vi "CRYSet RTA Front Panel.vi"(11 "Vi Ref in":refnum<vi> caption="Vi Ref") -> (3 "Vi Ref out":refnum<vi> caption="Vi Ref")   [LabVIEW 2013]
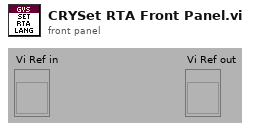
[diagram p1: front panel]
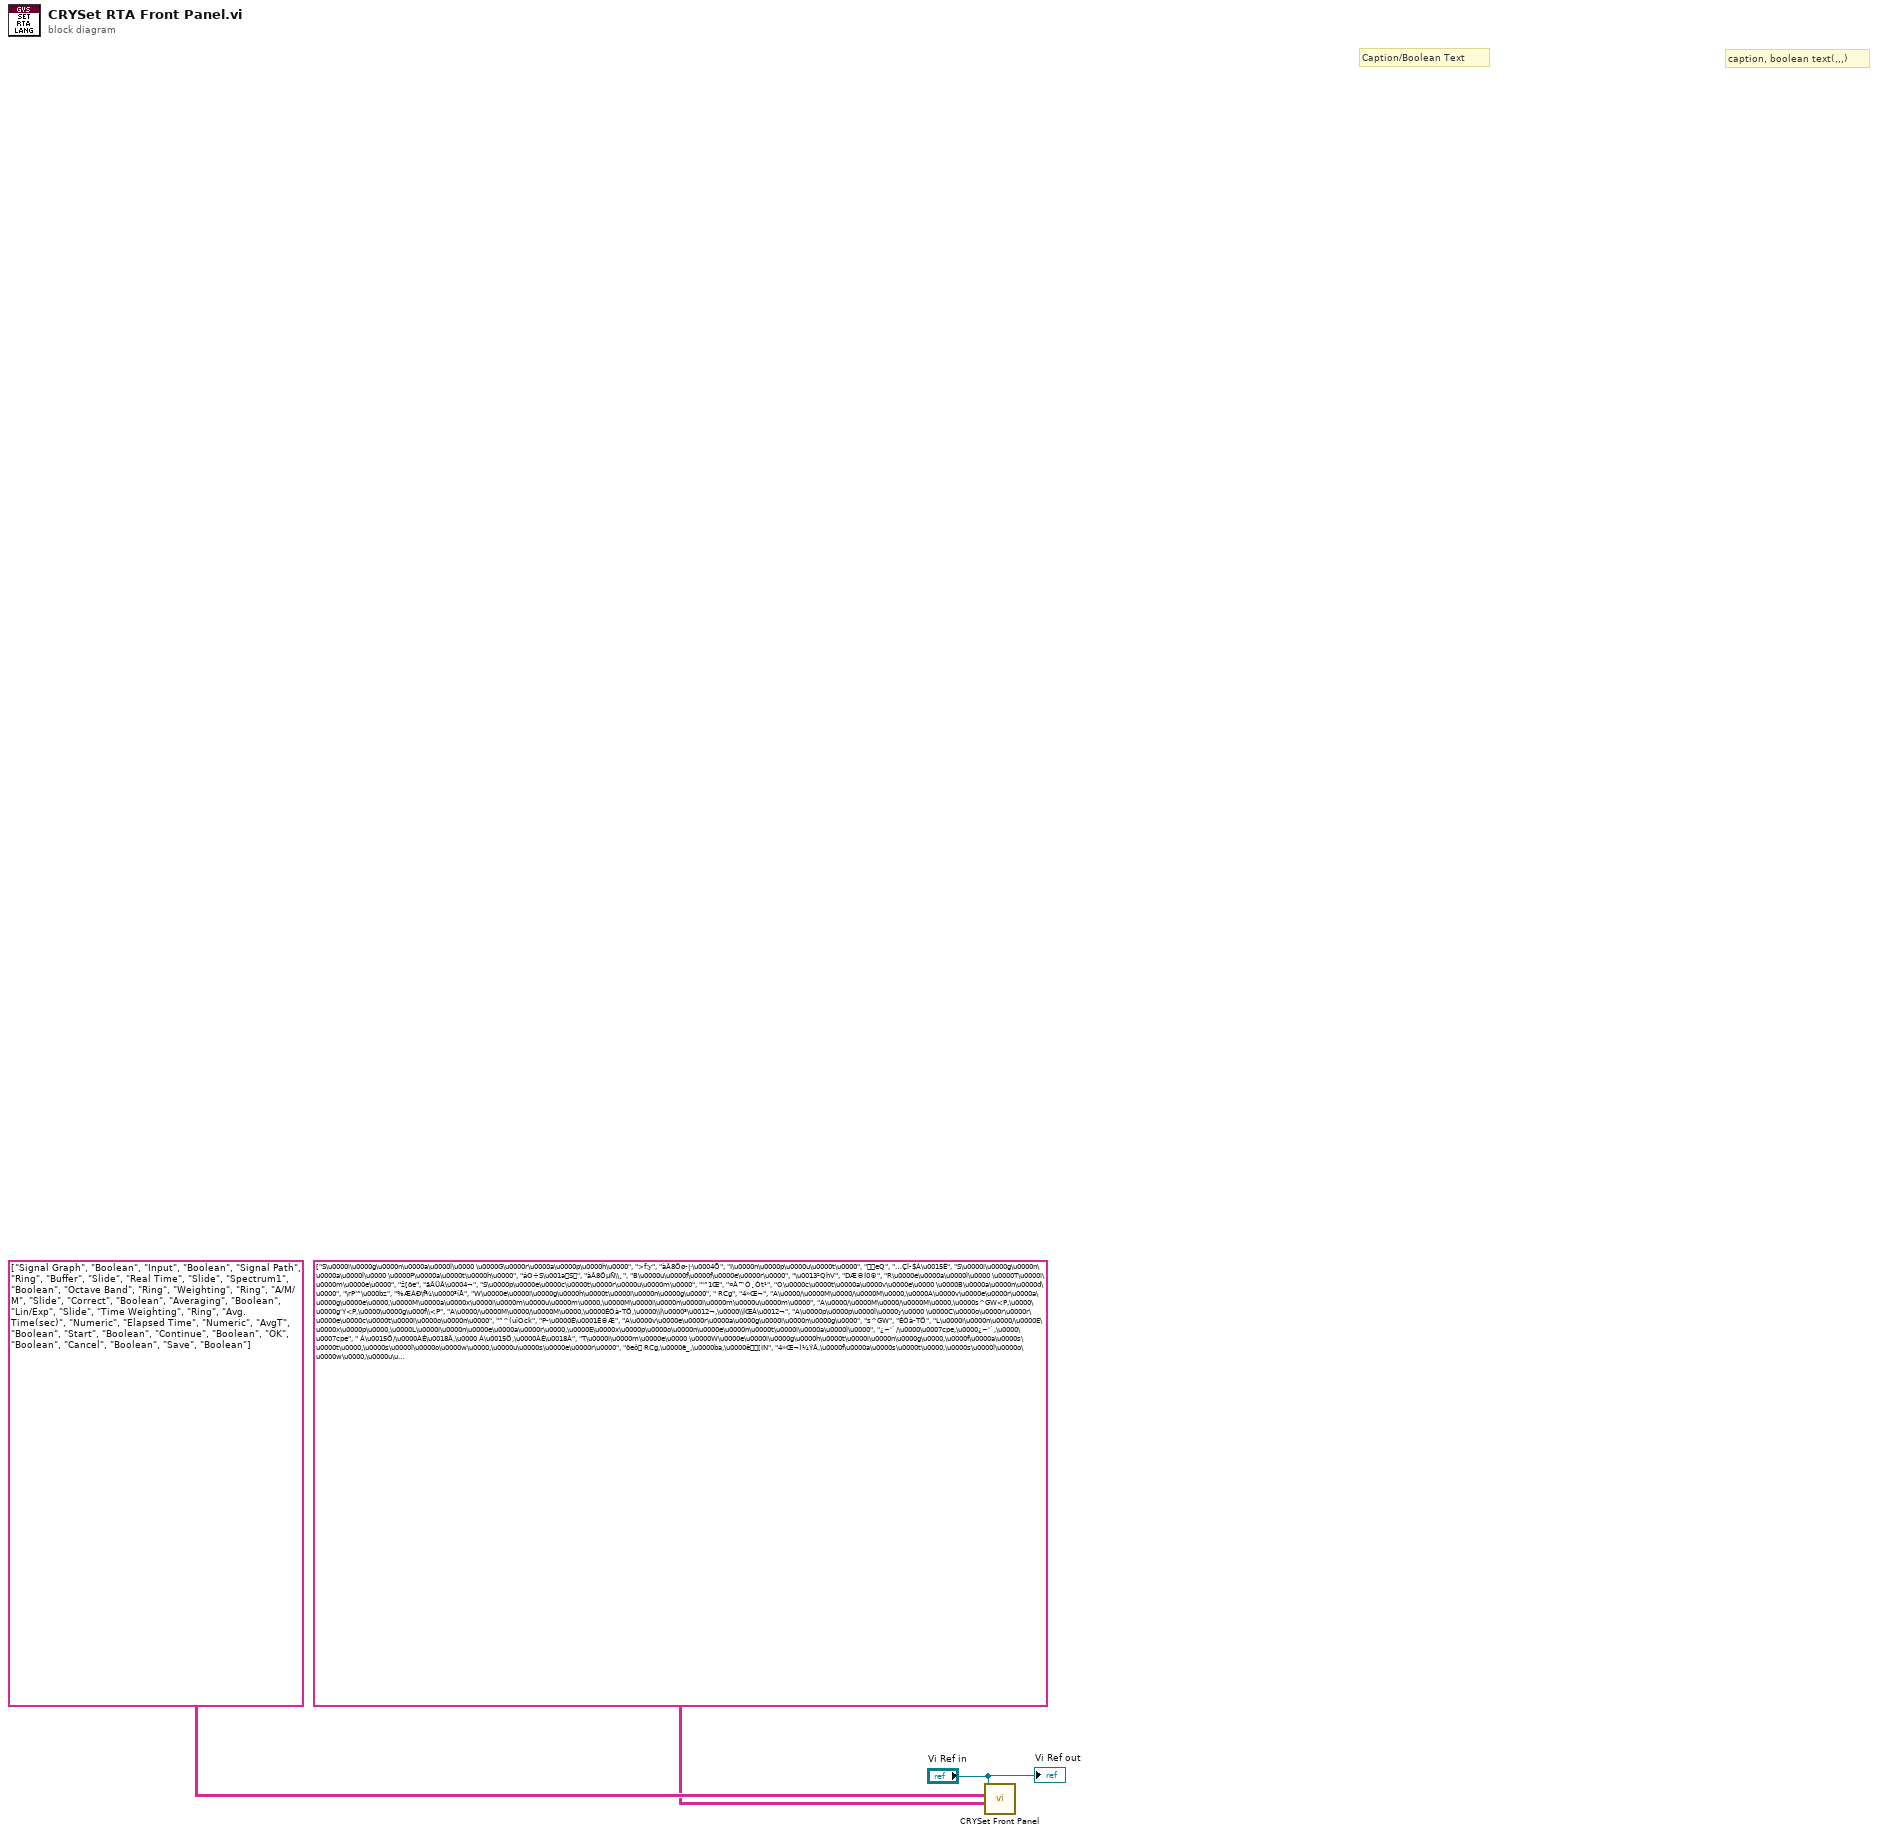
[diagram p0: block diagram]
diagram:
  # "caption, boolean text(,,,)"
  # "Caption/Boolean Text"
  n1 = call "CRYSet Front Panel.vi"("Caption(Boolean Text)"=string[][] [["S\u0000i\u0000g\u0000n\u0000a\u0000l\u0000 \u0000G\u0000r\u0000a\u0000p\u0000h\u0000", ">f:y", "àÂ8Öø­|·\u0004Õ"], ["I\u0000n\u0000p\u0000u\u0000t\u0000", "eQ", "…Çl­$Á\u0015È"], ["S\u0000i\u0000g\u0000n\u0000a\u0000l\u0000 \u0000P\u0000a\u0000t\u0000h\u0000", "áO÷S\u001aS", "àÂ8ÖµÑ\\¸"], ["B\u0000u\u0000f\u0000f\u0000e\u0000r\u0000", "\u0013²QhV", "DÆ©Í0®"], ["R\u0000e\u0000a\u0000l\u0000 \u0000T\u0000i\u0000m\u0000e\u0000", "ž[öe", "äÂÜÂ\u0004¬"], ["S\u0000p\u0000e\u0000c\u0000t\u0000r\u0000u\u0000m\u0000", "‘˜1Œ", "¤Â™Ó¸Òt¹"], ["O\u0000c\u0000t\u0000a\u0000v\u0000e\u0000 \u0000B\u0000a\u0000n\u0000d\u0000", "\rP‘˜\u000bz", "%ÆÀÐ\f¾\u0000³íÅ"], ["W\u0000e\u0000i\u0000g\u0000h\u0000t\u0000i\u0000n\u0000g\u0000", " RCg", "4»Œ¬"], ["A\u0000/\u0000M\u0000/\u0000M\u0000,\u0000A\u0000v\u0000e\u0000r\u0000a\u0000g\u0000e\u0000,\u0000M\u0000a\u0000x\u0000i\u0000m\u0000u\u0000m\u0000,\u0000M\u0000i\u0000n\u0000i\u0000m\u0000u\u0000m\u0000", "A\u0000/\u0000M\u0000/\u0000M\u0000,\u0000s^GW<P,\u0000\u0000g'Y<P,\u0000\u0000g\u000f\\<P", "A\u0000/\u0000M\u0000/\u0000M\u0000,\u0000ÉÓà­TÖ,\u0000\\Í\u0000³\u0012¬,\u0000\\ÍŒÁ\u0012¬"], ["A\u0000p\u0000p\u0000l\u0000y\u0000 \u0000C\u0000o\u0000r\u0000r\u0000e\u0000c\u0000t\u0000i\u0000o\u0000n\u0000", "”^(uîOck", "P­\u0000É\u0001È©Æ"], ["A\u0000v\u0000e\u0000r\u0000a\u0000g\u0000i\u0000n\u0000g\u0000", "s^GW", "ÉÓà­TÖ"], ["L\u0000i\u0000n\u0000/\u0000E\u0000x\u0000p\u0000,\u0000L\u0000i\u0000n\u0000e\u0000a\u0000r\u0000,\u0000E\u0000x\u0000p\u0000o\u0000n\u0000e\u0000n\u0000t\u0000i\u0000a\u0000l\u0000", "¿~'`/\u0000\u0007cpe,\u0000¿~'`,\u0000\u0007cpe", " Á\u0015Ö/\u0000ÀÉ\u0018Â,\u0000 Á\u0015Ö,\u0000ÀÉ\u0018Â"], ["T\u0000i\u0000m\u0000e\u0000 \u0000W\u0000e\u0000i\u0000g\u0000h\u0000t\u0000i\u0000n\u0000g\u0000,\u0000f\u0000a\u0000s\u0000t\u0000,\u0000s\u0000l\u0000o\u0000w\u0000,\u0000u\u0000s\u0000e\u0000r\u0000", "öeô RCg,\u0000ë_,\u0000ba,\u0000ê[IN", "4»Œ¬)¼ÝÂ,\u0000f\u0000a\u0000s\u0000t\u0000,\u0000s\u0000l\u0000o\u0000w\u0000,\u0000u\u0000s\u0000e\u0000r\u0000"], ["A\u0000v\u0000g\u0000.\u0000 \u0000T\u0000i\u0000m\u0000e\u0000(\u0000s\u0000e\u0000c\u0000)\u0000", "s^GWöeô•(\u0000Òy)\u0000", "ÉÓà­ÜÂ\u0004¬(\u0000\bÍ)\u0000"], ["E\u0000l\u0000a\u0000p\u0000s\u0000e\u0000d\u0000 \u0000T\u0000i\u0000m\u0000e\u0000", "ˆm\u0017€öeô•", "½¬ü¬ÜÂ\u0004¬"], ["A\u0000v\u0000e\u0000r\u0000a\u0000g\u0000i\u0000n\u0000g\u0000", "s^GW.\u0000.\u0000.\u0000", "ÉÓà­.\u0000.\u0000.\u0000"], ["S\u0000t\u0000a\u0000r\u0000t\u0000", "\u0000_ \u0000ËY", "ÜÂ \u0000‘Ç"], ["C\u0000o\u0000n\u0000t\u0000i\u0000n\u0000u\u0000e\u0000", "ç~ \u0000í~", "Ä¬ \u0000Á"], ["O\u0000K\u0000", "nx¤‹", "UÖxÇ"], ["C\u0000a\u0000n\u0000c\u0000e\u0000l\u0000", "ÖSˆm", "èÍŒÁ"], ["S\u0000a\u0000v\u0000e\u0000 \u0000t\u0000o\u0000 \u0000 \u0000C\u0000u\u0000r\u0000v\u0000e\u0000L\u0000i\u0000b\u0000", "ÝOX[0Ròf¿~“^", "á¬ Á\u001cÁà¬ÐÅ \u0000ô¼\u0000­"]], "Control ID and Type(Label Name, Type)"=string[][] [["Signal Graph", "Boolean"], ["Input", "Boolean"], ["Signal Path", "Ring"], ["Buffer", "Slide"], ["Real Time", "Slide"], ["Spectrum1", "Boolean"], ["Octave Band", "Ring"], ["Weighting", "Ring"], ["A/M/M", "Slide"], ["Correct", "Boolean"], ["Averaging", "Boolean"], ["Lin/Exp", "Slide"], ["Time Weighting", "Ring"], ["Avg. Time(sec)", "Numeric"], ["Elapsed Time", "Numeric"], ["AvgT", "Boolean"], ["Start", "Boolean"], ["Continue", "Boolean"], ["OK", "Boolean"], ["Cancel", "Boolean"], ["Save", "Boolean"]], "Vi Ref"="Vi Ref in") -> ()  [unwired: 9 in]
  "Vi Ref out" <- "Vi Ref in"
